vi "Global 1.vi"() -> ()   [LabVIEW 2015]
panel:
  in  "A_resister":dbl
  in  "A_sensor":string(combo)
  in  "Vac_pressure":dbl
  out "Boolean":bool
  in  "stop":bool
  in  "Time":string
  in  "Numeric 5":dbl
  in  "Sep_pressure":dbl
  in  "Sep_Flow":dbl
  in  "He3_pressure":dbl
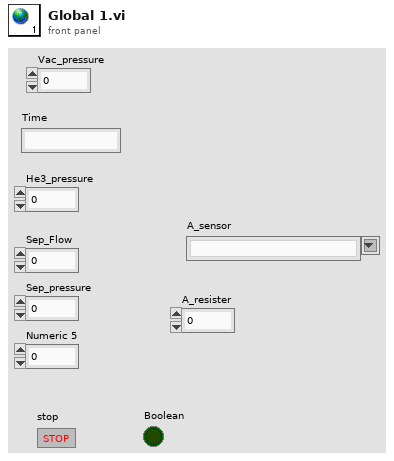
[diagram p1: front panel]
diagram:
